vi "Parse Character Set.vi"(10 "Numeric(2)":u16) -> (2 "DataTypes":T1)   [LabVIEW 2014, in "hse-db.lvlib" / "MySQL (TCP).lvlib"]
uses:
  MySQL (TCP).lvlib
  Controls/Character Set.ctl
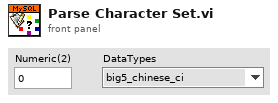
[diagram p1: front panel]
types:
  T1 = typedef "hse-db.lvlib/MySQL (TCP).lvlib/Character Set.ctl" = enum16{"big5_chinese_ci", "dec8_swedish_ci", "cp850_general_ci", "hp8_english_ci", "koi8r_general_ci", "latin1_swedish_ci", "latin2_general_ci", "swe7_swedish_ci", "ascii_general_ci", "ujis_japanese_ci", "sjis_japanese_ci", "hebrew_general_ci", "tis620_thai_ci", "euckr_korean_ci", "koi8u_general_ci", "gb2312_chinese_ci", "greek_general_ci", "cp1250_general_ci", "gbk_chinese_ci", "latin5_turkish_ci", "armscii8_general_ci", "utf8_general_ci", "ucs2_general_ci", "cp866_general_ci", "keybcs2_general_ci", "macce_general_ci", "macroman_general_ci", "cp852_general_ci", "latin7_general_ci", "cp1251_general_ci", "utf16_general_ci", "utf16le_general_ci", "cp1256_general_ci", "cp1257_general_ci", "utf32_general_ci", "binary", "geostd8_general_ci", "cp932_japanese_ci", "eucjpms_japanese_ci", "gb18030_chinese_ci", "utf8mb4_0900_ai_ci"}
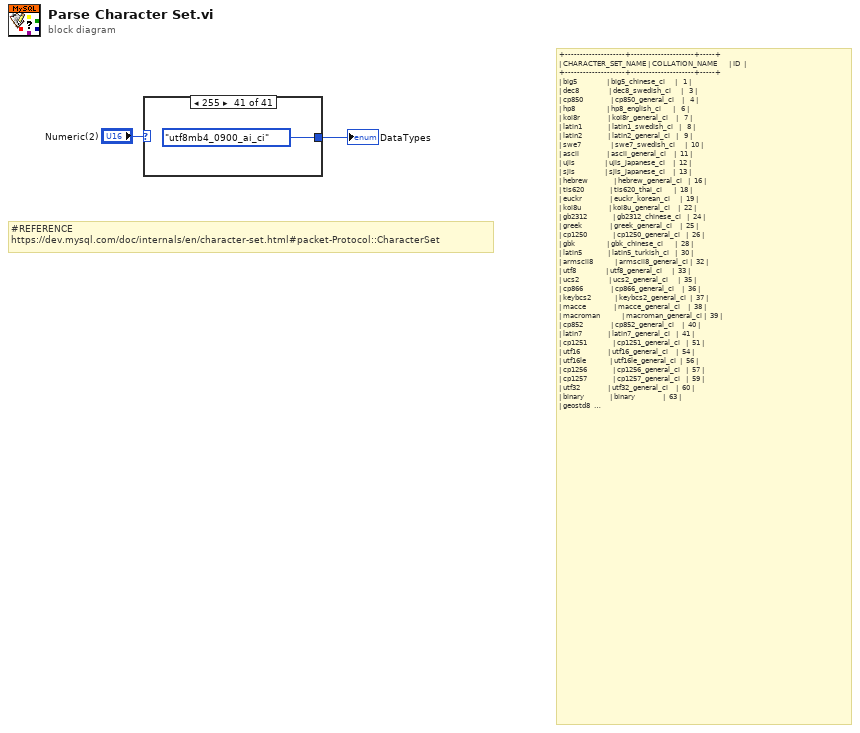
[diagram p0: block diagram]
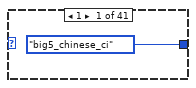
[diagram p2: hidden frame]
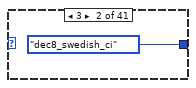
[diagram p3: hidden frame]
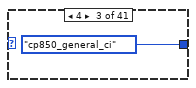
[diagram p4: hidden frame]
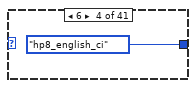
[diagram p5: hidden frame]
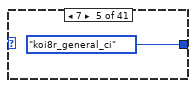
[diagram p6: hidden frame]
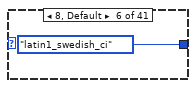
[diagram p7: hidden frame]
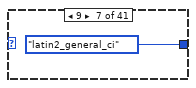
[diagram p8: hidden frame]
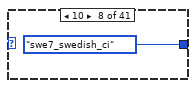
[diagram p9: hidden frame]
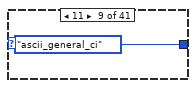
[diagram p10: hidden frame]
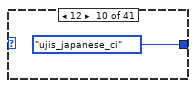
[diagram p11: hidden frame]
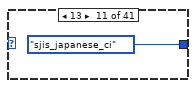
[diagram p12: hidden frame]
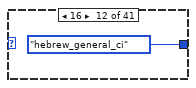
[diagram p13: hidden frame]
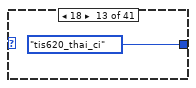
[diagram p14: hidden frame]
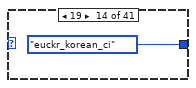
[diagram p15: hidden frame]
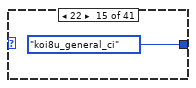
[diagram p16: hidden frame]
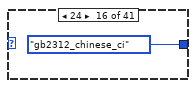
[diagram p17: hidden frame]
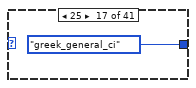
[diagram p18: hidden frame]
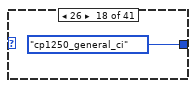
[diagram p19: hidden frame]
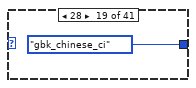
[diagram p20: hidden frame]
diagram:
  # "+--------------------+---------------------+-----+\n| CHARACTER_SET_NAME | COLLATION_NAME      | ID  |\n+--------------------+---------------------+-----+\n| big5               | big5_chinese_ci     |   1 |\n| dec8               | dec8_swedish_ci     |   3 |\n| cp850              | cp850_general_ci    |   4 |\n| hp8                | hp8_english_ci      |   6 |\n| koi8r              | koi8r_general_ci    |   7 |\n| latin1             | latin1_swedish_ci   |   8 |\n| latin2             | latin2_general_ci   |   9 |\n| swe7               | swe7_swedish_ci     |  10 |\n| ascii              | ascii_general_ci    |  11 |\n| ujis               | ujis_japanese_ci    |  12 |\n| sjis               | sjis_japanese_ci    |  13 |\n| hebrew             | hebrew_general_ci   |  16 |\n| tis620             | tis620_thai_ci      |  18 |\n| euckr              | euckr_korean_ci     |  19 |\n| koi8u              | koi8u_general_ci    |  22 |\n| gb2312             | gb2312_chinese_ci   |  24 |\n| greek              | greek_general_ci    |  25 |\n| cp1250             | cp1250_general_ci   |  26 |\n| gbk                | gbk_chinese_ci      |  28 |\n| latin5             | latin5_turkish_ci   |  30 |\n| armscii8           | armscii8_general_ci |  32 |\n| utf8               | utf8_general_ci     |  33 |\n| ucs2               | ucs2_general_ci     |  35 |\n| cp866              | cp866_general_ci    |  36 |\n| keybcs2            | keybcs2_general_ci  |  37 |\n| macce              | macce_general_ci    |  38 |\n| macroman           | macroman_general_ci |  39 |\n| cp852              | cp852_general_ci    |  40 |\n| latin7             | latin7_general_ci   |  41 |\n| cp1251             | cp1251_general_ci   |  51 |\n| utf16              | utf16_general_ci    |  54 |\n| utf16le            | utf16le_general_ci  |  56 |\n| cp1256             | cp1256_general_ci   |  57 |\n| cp1257             | cp1257_general_ci   |  59 |\n| utf32              | utf32_general_ci    |  60 |\n| binary             | binary              |  63 |\n| geostd8            | geostd8_general_ci  |  92 |\n| cp932              | cp932_japanese_ci   |  95 |\n| eucjpms            | eucjpms_japanese_ci |  97 |\n| gb18030            | gb18030_chinese_ci  | 248 |\n| utf8mb4            | utf8mb4_0900_ai_ci  | 255 |\n+--------------------+---------------------+-----+"
  # "#REFERENCE\nhttps://dev.mysql.com/doc/internals/en/character-set.html#packet-Protocol::CharacterSet"
  n1 = case shown="255" "Numeric(2)" {
    tunnel: [Character_Set."big5_chinese_ci" ("MySQLDataTypes") Character_Set."dec8_swedish_ci" ("MySQLDataTypes") Character_Set."cp850_general_ci" ("MySQLDataTypes") Character_Set."hp8_english_ci" ("MySQLDataTypes") Character_Set."koi8r_general_ci" ("MySQLDataTypes") Character_Set."latin1_swedish_ci" ("MySQLDataTypes") Character_Set."latin2_general_ci" ("MySQLDataTypes") Character_Set."swe7_swedish_ci" ("MySQLDataTypes") Character_Set."ascii_general_ci" ("MySQLDataTypes") Character_Set."ujis_japanese_ci" ("MySQLDataTypes") Character_Set."sjis_japanese_ci" ("MySQLDataTypes") Character_Set."hebrew_general_ci" ("MySQLDataTypes") Character_Set."tis620_thai_ci" ("MySQLDataTypes") Character_Set."euckr_korean_ci" ("MySQLDataTypes") Character_Set."koi8u_general_ci" ("MySQLDataTypes") Character_Set."gb2312_chinese_ci" ("MySQLDataTypes") Character_Set."greek_general_ci" ("MySQLDataTypes") Character_Set."cp1250_general_ci" ("MySQLDataTypes") Character_Set."gbk_chinese_ci" ("MySQLDataTypes") Character_Set."latin5_turkish_ci" ("MySQLDataTypes") Character_Set."armscii8_general_ci" ("MySQLDataTypes") Character_Set."utf8_general_ci" ("MySQLDataTypes") Character_Set."ucs2_general_ci" ("MySQLDataTypes") Character_Set."cp866_general_ci" ("MySQLDataTypes") Character_Set."keybcs2_general_ci" ("MySQLDataTypes") Character_Set."macce_general_ci" ("MySQLDataTypes") Character_Set."macroman_general_ci" ("MySQLDataTypes") Character_Set."cp852_general_ci" ("MySQLDataTypes") Character_Set."latin7_general_ci" ("MySQLDataTypes") Character_Set."cp1251_general_ci" ("MySQLDataTypes") Character_Set."utf16_general_ci" ("MySQLDataTypes") Character_Set."utf16le_general_ci" ("MySQLDataTypes") Character_Set."cp1256_general_ci" ("MySQLDataTypes") Character_Set."cp1257_general_ci" ("MySQLDataTypes") Character_Set."utf32_general_ci" ("MySQLDataTypes") Character_Set."binary" ("MySQLDataTypes") Character_Set."geostd8_general_ci" ("MySQLDataTypes") Character_Set."cp932_japanese_ci" ("MySQLDataTypes") Character_Set."eucjpms_japanese_ci" ("MySQLDataTypes") Character_Set."gb18030_chinese_ci" ("MySQLDataTypes") Character_Set."utf8mb4_0900_ai_ci" ("MySQLDataTypes")] -> w1
    frame 1 {
    }
    frame 3 {
    }
    frame 4 {
    }
    frame 6 {
    }
    frame 7 {
    }
    frame 8, Default {
    }
    frame 9 {
    }
    frame 10 {
    }
    frame 11 {
    }
    frame 12 {
    }
    frame 13 {
    }
    frame 16 {
    }
    frame 18 {
    }
    frame 19 {
    }
    frame 22 {
    }
    frame 24 {
    }
    frame 25 {
    }
    frame 26 {
    }
    frame 28 {
    }
    frame 30 {
    }
    frame 32 {
    }
    frame 33 {
    }
    frame 35 {
    }
    frame 36 {
    }
    frame 37 {
    }
    frame 38 {
    }
    frame 39 {
    }
    frame 40 {
    }
    frame 41 {
    }
    frame 51 {
    }
    frame 54 {
    }
    frame 56 {
    }
    frame 57 {
    }
    frame 59 {
    }
    frame 60 {
    }
    frame 63 {
    }
    frame 92 {
    }
    frame 95 {
    }
    frame 97 {
    }
    frame 248 {
    }
    frame 255 {
    }
  }
  "DataTypes" <- w1
